vi "output.vi"(8 "error in":errorcluster, 10 "data table in":T1, 11 "OPC UA runtime in":refnum<class "OPC UA runtime.lvclass">) -> (0 "error out":errorcluster, 2 "data table out":T1, 3 "OPC UA runtime out":refnum<class "OPC UA runtime.lvclass">)   [LabVIEW 2013, in "OPC UA runtime.lvclass"]
doc: "Provides an interface for writing data to a module at runtime. While this interface performs no operations, a child should provide an override which may write to any open sessions, references, or interfaces."
uses:
  OPC UA runtime.lvclass
  <vilib>/NI/Tag Bus/table/data table.lvlib
  <vilib>/NI/Tag Bus/table/data polymorphs/read one/read Boolean.vi
  <vilib>/opcua/NI OPC UA Client.lvlib
  <vilib>/OPCUA/client/Write Bool.vi
  <vilib>/NI/Tag Bus/table/data polymorphs/read one/read I8.vi
  <vilib>/OPCUA/client/Write SByte.vi
  <vilib>/NI/Tag Bus/table/data polymorphs/read one/read U8.vi
  <vilib>/OPCUA/client/Write Byte.vi
  <vilib>/OPCUA/client/Write Int16.vi
  <vilib>/NI/Tag Bus/table/data polymorphs/read one/read I16.vi
  <vilib>/OPCUA/client/Write UInt16.vi
  <vilib>/NI/Tag Bus/table/data polymorphs/read one/read U16.vi
  <vilib>/OPCUA/client/Write Int32.vi
  <vilib>/NI/Tag Bus/table/data polymorphs/read one/read I32.vi
  <vilib>/OPCUA/client/Write UInt32.vi
  <vilib>/NI/Tag Bus/table/data polymorphs/read one/read U32.vi
  <vilib>/OPCUA/client/Write Int64.vi
  <vilib>/NI/Tag Bus/table/data polymorphs/read one/read I64.vi
  <vilib>/OPCUA/client/Write UInt64.vi
  <vilib>/NI/Tag Bus/table/data polymorphs/read one/read U64.vi
  <vilib>/OPCUA/client/Write Float.vi
  <vilib>/NI/Tag Bus/table/data polymorphs/read one/read Single.vi
  <vilib>/OPCUA/client/Write Double.vi
  <vilib>/NI/Tag Bus/table/data polymorphs/read one/read Double.vi
  <vilib>/OPCUA/client/Write String.vi
  <vilib>/NI/Tag Bus/table/data polymorphs/read one/read String.vi
  <vilib>/OPCUA/client/Write DateTime.vi
  <vilib>/OPCUA/client/Write ByteString.vi
  <vilib>/NI/Tag Bus/table/data polymorphs/read one/read Array of U8.vi
  <vilib>/OPCUA/client/Write Bool Array.vi
  <vilib>/NI/Tag Bus/table/data polymorphs/read one/read Array of Boolean.vi
  <vilib>/NI/Tag Bus/table/data polymorphs/read one/read Array of I8.vi
  <vilib>/OPCUA/client/Write SByte Array.vi
  <vilib>/OPCUA/client/Write Byte Array.vi
  <vilib>/OPCUA/client/Write Int16 Array.vi
  <vilib>/NI/Tag Bus/table/data polymorphs/read one/read Array of I16.vi
  <vilib>/OPCUA/client/Write UInt16 Array.vi
  <vilib>/NI/Tag Bus/table/data polymorphs/read one/read Array of U16.vi
  <vilib>/OPCUA/client/Write Int32 Array.vi
  <vilib>/NI/Tag Bus/table/data polymorphs/read one/read Array of I32.vi
  <vilib>/OPCUA/client/Write UInt32 Array.vi
  <vilib>/NI/Tag Bus/table/data polymorphs/read one/read Array of U32.vi
  <vilib>/OPCUA/client/Write Int64 Array.vi
  <vilib>/NI/Tag Bus/table/data polymorphs/read one/read Array of I64.vi
  <vilib>/OPCUA/client/Write UInt64 Array.vi
  <vilib>/NI/Tag Bus/table/data polymorphs/read one/read Array of U64.vi
  <vilib>/OPCUA/client/Write Float Array.vi
  <vilib>/NI/Tag Bus/table/data polymorphs/read one/read Array of Single.vi
  <vilib>/OPCUA/client/Write Double Array.vi
  <vilib>/NI/Tag Bus/table/data polymorphs/read one/read Array of Double.vi
  <vilib>/OPCUA/client/Write String Array.vi
  <vilib>/NI/Tag Bus/table/data polymorphs/read one/read Array of String.vi
  <vilib>/OPCUA/client/Write DateTime Array.vi
  <vilib>/OPCUA/client/Write ByteString Array.vi
  <vilib>/opcua/NI OPC UA Server.lvlib
  <vilib>/OPCUA/server/Write Bool.vi
  <vilib>/OPCUA/server/Write SByte.vi
  <vilib>/OPCUA/server/Write Byte.vi
  <vilib>/OPCUA/server/Write Int16.vi
  <vilib>/OPCUA/server/Write UInt16.vi
  <vilib>/OPCUA/server/Write Int32.vi
  <vilib>/OPCUA/server/Write UInt32.vi
  <vilib>/OPCUA/server/Write Int64.vi
  <vilib>/OPCUA/server/Write UInt64.vi
  <vilib>/OPCUA/server/Write Float.vi
  <vilib>/OPCUA/server/Write Double.vi
  <vilib>/OPCUA/server/Write String.vi
  <vilib>/OPCUA/server/Write Date Time.vi
  <vilib>/OPCUA/server/Write Byte String.vi
  <vilib>/OPCUA/server/Write Bool Array.vi
  <vilib>/OPCUA/server/Write SByte Array.vi
  <vilib>/OPCUA/server/Write Byte Array.vi
  <vilib>/OPCUA/server/Write Int16 Array.vi
  <vilib>/OPCUA/server/Write UInt16 Array.vi
  <vilib>/OPCUA/server/Write Int32 Array.vi
  <vilib>/OPCUA/server/Write UInt32 Array.vi
  <vilib>/OPCUA/server/Write Int64 Array.vi
  <vilib>/OPCUA/server/Write UInt64 Array.vi
  <vilib>/OPCUA/server/Write Float Array.vi
  <vilib>/OPCUA/server/Write Double Array.vi
  <vilib>/OPCUA/server/Write String Array.vi
  <vilib>/OPCUA/server/Write Date Time Array.vi
  <vilib>/OPCUA/server/Write Byte String Array.vi
  <vilib>/NI/Tag Bus/table/data table.ctl
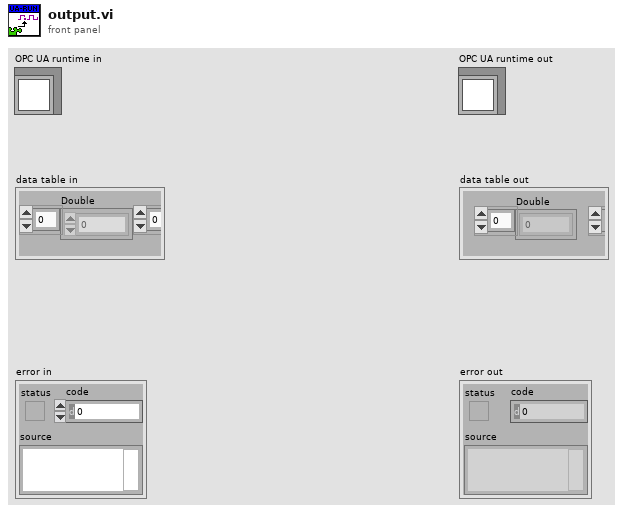
[diagram p1: front panel]
types:
  T1 = typedef "tag bus.lvlib/data table.lvlib/data table.ctl" = cluster{"Double":dbl[], "Single":sgl[], "I64":i64[], "I32":i32[], "I16":i16[], "I8":i8[], "U64":u64[], "U32":u32[], "U16":u16[], "U8":u8[], "Boolean":bool[], "String":string[], "Array of Double":cluster{"DBL Array":dbl[]}[], "Array of Single":cluster{"SGL Array":sgl[]}[], "Array of I64":cluster{"I64 Array":i64[]}[], "Array of I32":cluster{"I32 Array":i32[]}[], "Array of I16":cluster{"I16 Array":i16[]}[], "Array of I8":cluster{"I8 Array":i8[]}[], "Array of U64":cluster{"U64 Array":u64[]}[], "Array of U32":cluster{"U32 Array":u32[]}[], "Array of U16":cluster{"U16 Array":u16[]}[], "Array of U8":cluster{"U8 Array":u8[]}[], "Array of Boolean":cluster{"Boolean Array":bool[]}[], "Array of String":cluster{"String Array":string[]}[]}
  T2 = typedef "tag bus.lvlib/tag descriptor.lvclass/Data Type.ctl" = enum16{"Double", "Single", "I64", "I32", "I16", "I8", "U64", "U32", "U16", "U8", "Boolean", "String", "Array of Double", "Array of Single", "Array of I64", "Array of I32", "Array of I16", "Array of I8", "Array of U64", "Array of U32", "Array of U16", "Array of U8", "Array of Boolean", "Array of String"}
  T3 = typedef "OPC UA configuration.lvclass/OPC UA Data Type.ctl" = u16
  T4 = cluster{"DCAF Data Type":T2, "Index":i32, "Node Path":string, "OPC UA Data Type":T3}[]
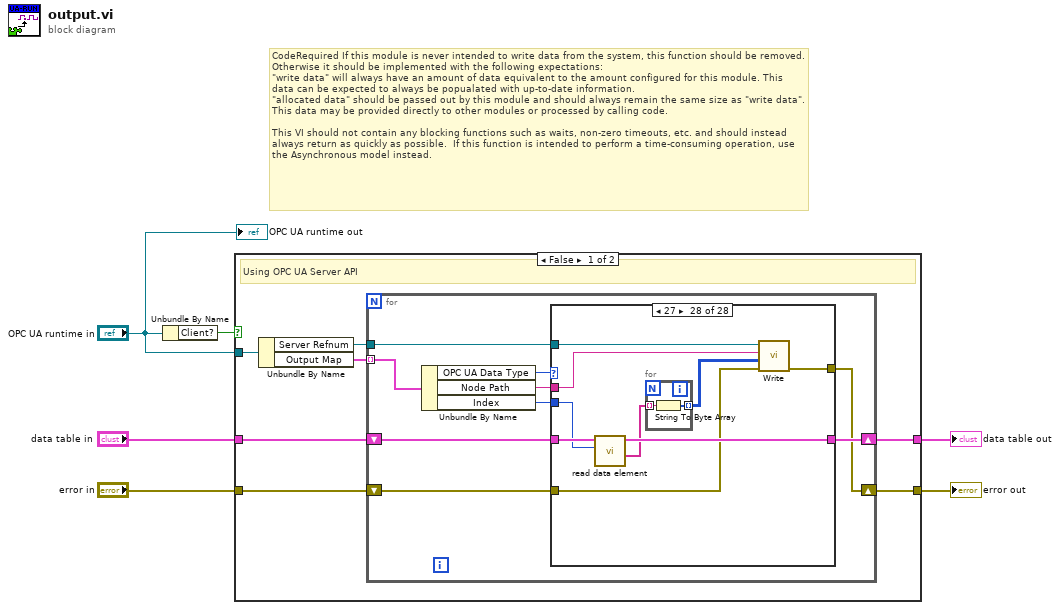
[diagram p0: block diagram]
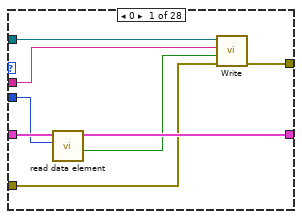
[diagram p2: hidden frame]
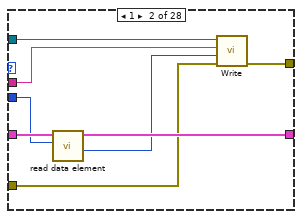
[diagram p3: hidden frame]
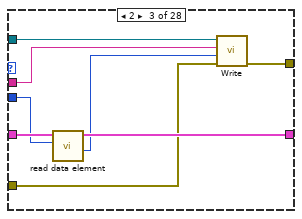
[diagram p4: hidden frame]
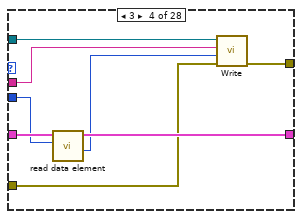
[diagram p5: hidden frame]
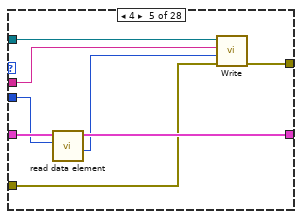
[diagram p6: hidden frame]
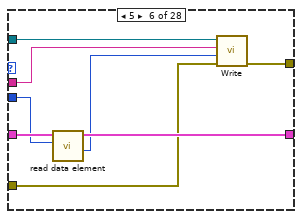
[diagram p7: hidden frame]
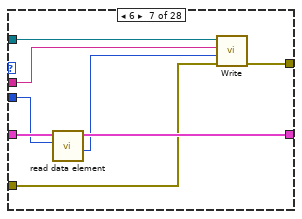
[diagram p8: hidden frame]
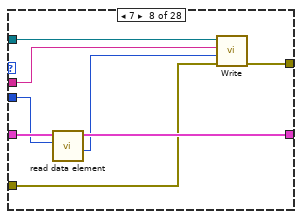
[diagram p9: hidden frame]
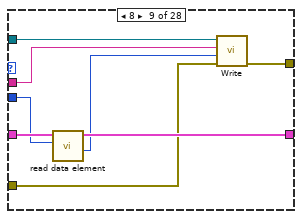
[diagram p10: hidden frame]
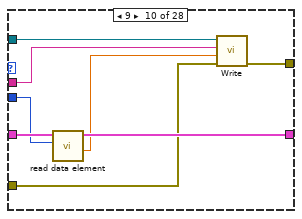
[diagram p11: hidden frame]
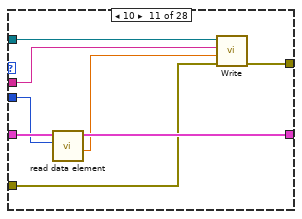
[diagram p12: hidden frame]
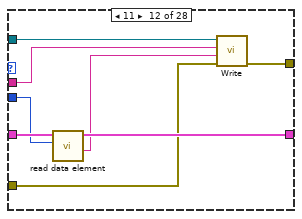
[diagram p13: hidden frame]
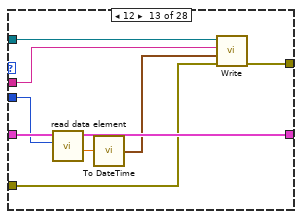
[diagram p14: hidden frame]
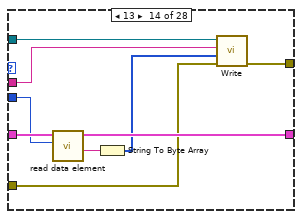
[diagram p15: hidden frame]
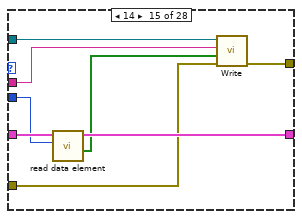
[diagram p16: hidden frame]
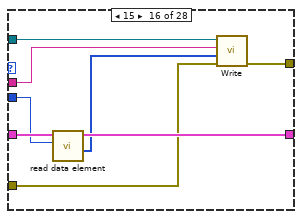
[diagram p17: hidden frame]
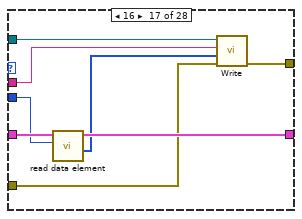
[diagram p18: hidden frame]
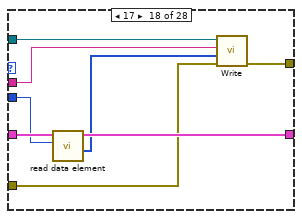
[diagram p19: hidden frame]
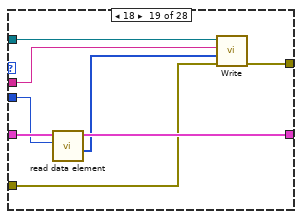
[diagram p20: hidden frame]
diagram:
  # "CodeRequired If this module is never intended to write data from the system, this function should be removed. Otherwise it should be implemented with the following expectations:\n\"write data\" will always have an amount of data equivalent to the amount configured for this module. This data can be expected to always be popualated with up-to-date information.\n\"allocated data\" should be passed out by this module and should always remain the same size as \"write data\". This data may be provided directly to other modules or processed by calling code.\n\nThis VI should not contain any blocking functions such as waits, non-zero timeouts, etc. and should instead always return as quickly as possible.  If this function is intended to perform a time-consuming operation, use the Asynchronous model instead."
  n1 = Unbundle By Name("OPC UA runtime in") -> ("Client?"=w6:bool)
  n2 = case shown="False" w6 {
    tunnel: "OPC UA runtime in" -> [w13 w259]
    tunnel: "data table in" -> [w9 w256]
    tunnel: "error in" -> [w8 w255]
    tunnel: [w10 w254] -> w2
    tunnel: [w7 w253] -> w3
    frame False {
      # "Using OPC UA Server API"
      n3 = Unbundle By Name(w13) -> ("Server Refnum"=w11:refnum<k21>, "Output Map"=w12:T4)
      n4 = for {
        tunnel: w11 -> [w16]
        tunnel: w12 -> [w22] mode=indexing
        shift-right: [w15] -> w7
        shift-left: w8 -> [w18]
        shift-right: [w19] -> w10
        shift-left: w9 -> [w20]
        n5 = Unbundle By Name(w22) -> ("OPC UA Data Type"=w21:T3, "Node Path"=w14:string, "Index"=w17:i32)
        n6 = case shown="27" w21 {
          tunnel: w20 -> [w30 w38 w46 w54 w62 w70 w78 w86 w94 w102 w110 w118 w127 w136 w144 w152 w160 w168 w176 w184 w192 w200 w208 w216 w224 w232 w241 w250]
          tunnel: [w29 w37 w45 w53 w61 w69 w77 w85 w93 w101 w109 w117 w126 w135 w143 w151 w159 w167 w175 w183 w191 w199 w207 w215 w223 w231 w240 w249] -> w19
          tunnel: w18 -> [w25 w33 w41 w49 w57 w65 w73 w81 w89 w97 w105 w113 w122 w131 w139 w147 w155 w163 w171 w179 w187 w195 w203 w211 w219 w227 w236 w245]
          tunnel: w17 -> [w28 w36 w44 w52 w60 w68 w76 w84 w92 w100 w108 w116 w125 w134 w142 w150 w158 w166 w174 w182 w190 w198 w206 w214 w222 w230 w239 w248]
          tunnel: w16 -> [w27 w35 w43 w51 w59 w67 w75 w83 w91 w99 w107 w115 w124 w133 w141 w149 w157 w165 w173 w181 w189 w197 w205 w213 w221 w229 w238 w247]
          tunnel: [w26 w34 w42 w50 w58 w66 w74 w82 w90 w98 w106 w114 w123 w132 w140 w148 w156 w164 w172 w180 w188 w196 w204 w212 w220 w228 w237 w246] -> w15
          tunnel: w14 -> [w24 w32 w40 w48 w56 w64 w72 w80 w88 w96 w104 w112 w121 w130 w138 w146 w154 w162 w170 w178 w186 w194 w202 w210 w218 w226 w235 w244]
          frame 0 {
            n7 = call-poly <vilib>:"read data element.vi"("index"=w28, "data table in"=w30) -> ("value"=w23:bool, "data table out"=w29:T1)  [unwired: 8 in]
            n8 = call-poly <vilib>:"Write.vi"("error in (no error)"=w25, "value"=w23, "node path"=w24, "OPC UA server refnum in"=w27) -> ("error out"=w26:errorcluster)  [unwired: 6 in, 1 out]
          }
          frame 1 {
            n9 = call-poly <vilib>:"read data element.vi"("index"=w36, "data table in"=w38) -> ("value"=w31:i8, "data table out"=w37:T1)  [unwired: 8 in]
            n10 = call-poly <vilib>:"Write.vi"("error in (no error)"=w33, "value"=w31, "node path"=w32, "OPC UA server refnum in"=w35) -> ("error out"=w34:errorcluster)  [unwired: 6 in, 1 out]
          }
          frame 2 {
            n11 = call-poly <vilib>:"read data element.vi"("index"=w44, "data table in"=w46) -> ("value"=w39:u8, "data table out"=w45:T1)  [unwired: 8 in]
            n12 = call-poly <vilib>:"Write.vi"("error in (no error)"=w41, "value"=w39, "node path"=w40, "OPC UA server refnum in"=w43) -> ("error out"=w42:errorcluster)  [unwired: 6 in, 1 out]
          }
          frame 3 {
            n13 = call-poly <vilib>:"read data element.vi"("index"=w52, "data table in"=w54) -> ("value"=w47:i16, "data table out"=w53:T1)  [unwired: 8 in]
            n14 = call-poly <vilib>:"Write.vi"("error in (no error)"=w49, "value"=w47, "node path"=w48, "OPC UA server refnum in"=w51) -> ("error out"=w50:errorcluster)  [unwired: 6 in, 1 out]
          }
          frame 4 {
            n15 = call-poly <vilib>:"read data element.vi"("index"=w60, "data table in"=w62) -> ("value"=w55:u16, "data table out"=w61:T1)  [unwired: 8 in]
            n16 = call-poly <vilib>:"Write.vi"("error in (no error)"=w57, "value"=w55, "node path"=w56, "OPC UA server refnum in"=w59) -> ("error out"=w58:errorcluster)  [unwired: 6 in, 1 out]
          }
          frame 5 {
            n17 = call-poly <vilib>:"read data element.vi"("index"=w68, "data table in"=w70) -> ("value"=w63:i32, "data table out"=w69:T1)  [unwired: 8 in]
            n18 = call-poly <vilib>:"Write.vi"("error in (no error)"=w65, "value"=w63, "node path"=w64, "OPC UA server refnum in"=w67) -> ("error out"=w66:errorcluster)  [unwired: 6 in, 1 out]
          }
          frame 6 {
            n19 = call-poly <vilib>:"read data element.vi"("index"=w76, "data table in"=w78) -> ("value"=w71:u32, "data table out"=w77:T1)  [unwired: 8 in]
            n20 = call-poly <vilib>:"Write.vi"("error in (no error)"=w73, "value"=w71, "node path"=w72, "OPC UA server refnum in"=w75) -> ("error out"=w74:errorcluster)  [unwired: 6 in, 1 out]
          }
          frame 7 {
            n21 = call-poly <vilib>:"read data element.vi"("index"=w84, "data table in"=w86) -> ("value"=w79:i64, "data table out"=w85:T1)  [unwired: 8 in]
            n22 = call-poly <vilib>:"Write.vi"("error in (no error)"=w81, "value"=w79, "node path"=w80, "OPC UA server refnum in"=w83) -> ("error out"=w82:errorcluster)  [unwired: 6 in, 1 out]
          }
          frame 8 {
            n23 = call-poly <vilib>:"read data element.vi"("index"=w92, "data table in"=w94) -> ("value"=w87:u64, "data table out"=w93:T1)  [unwired: 8 in]
            n24 = call-poly <vilib>:"Write.vi"("error in (no error)"=w89, "value"=w87, "node path"=w88, "OPC UA server refnum in"=w91) -> ("error out"=w90:errorcluster)  [unwired: 6 in, 1 out]
          }
          frame 9 {
            n25 = call-poly <vilib>:"read data element.vi"("index"=w100, "data table in"=w102) -> ("value"=w95:sgl, "data table out"=w101:T1)  [unwired: 8 in]
            n26 = call-poly <vilib>:"Write.vi"("error in (no error)"=w97, "value"=w95, "node path"=w96, "OPC UA server refnum in"=w99) -> ("error out"=w98:errorcluster)  [unwired: 6 in, 1 out]
          }
          frame 10 {
            n27 = call-poly <vilib>:"read data element.vi"("index"=w108, "data table in"=w110) -> ("value"=w103:dbl, "data table out"=w109:T1)  [unwired: 8 in]
            n28 = call-poly <vilib>:"Write.vi"("error in (no error)"=w105, "value"=w103, "node path"=w104, "OPC UA server refnum in"=w107) -> ("error out"=w106:errorcluster)  [unwired: 6 in, 1 out]
          }
          frame 11 {
            n29 = call-poly <vilib>:"read data element.vi"("index"=w116, "data table in"=w118) -> ("value"=w111:string, "data table out"=w117:T1)  [unwired: 8 in]
            n30 = call-poly <vilib>:"Write.vi"("error in (no error)"=w113, "value"=w111, "node path"=w112, "OPC UA server refnum in"=w115) -> ("error out"=w114:errorcluster)  [unwired: 6 in, 1 out]
          }
          frame 12 {
            n31 = call-poly <vilib>:"read data element.vi"("index"=w125, "data table in"=w127) -> ("value"=w120:dbl, "data table out"=w126:T1)  [unwired: 8 in]
            n32 = call "To DateTime.vi"("Formatted DateTime"=w120) -> ("Time Stamp"=w119:timestamp)
            n33 = call-poly <vilib>:"Write.vi"("error in (no error)"=w122, "value"=w119, "node path"=w121, "OPC UA server refnum in"=w124) -> ("error out"=w123:errorcluster)  [unwired: 6 in, 1 out]
          }
          frame 13 {
            n34 = call-poly <vilib>:"read data element.vi"("index"=w134, "data table in"=w136) -> ("value"=w129:string, "data table out"=w135:T1)  [unwired: 8 in]
            n35 = String To Byte Array(string=w129) -> (unsigned byte array=w128:u8[])
            n36 = call-poly <vilib>:"Write.vi"("error in (no error)"=w131, "value"=w128, "node path"=w130, "OPC UA server refnum in"=w133) -> ("error out"=w132:errorcluster)  [unwired: 6 in, 1 out]
          }
          frame 14 {
            n37 = call-poly <vilib>:"read data element.vi"("index"=w142, "data table in"=w144) -> ("value"=w137:bool[], "data table out"=w143:T1)  [unwired: 8 in]
            n38 = call-poly <vilib>:"Write.vi"("error in (no error)"=w139, "value"=w137, "node path"=w138, "OPC UA server refnum in"=w141) -> ("error out"=w140:errorcluster)  [unwired: 6 in, 1 out]
          }
          frame 15 {
            n39 = call-poly <vilib>:"read data element.vi"("index"=w150, "data table in"=w152) -> ("value"=w145:i8[], "data table out"=w151:T1)  [unwired: 8 in]
            n40 = call-poly <vilib>:"Write.vi"("error in (no error)"=w147, "value"=w145, "node path"=w146, "OPC UA server refnum in"=w149) -> ("error out"=w148:errorcluster)  [unwired: 6 in, 1 out]
          }
          frame 16 {
            n41 = call-poly <vilib>:"read data element.vi"("index"=w158, "data table in"=w160) -> ("value"=w153:u8[], "data table out"=w159:T1)  [unwired: 8 in]
            n42 = call-poly <vilib>:"Write.vi"("error in (no error)"=w155, "value"=w153, "node path"=w154, "OPC UA server refnum in"=w157) -> ("error out"=w156:errorcluster)  [unwired: 6 in, 1 out]
          }
          frame 17 {
            n43 = call-poly <vilib>:"read data element.vi"("index"=w166, "data table in"=w168) -> ("value"=w161:i16[], "data table out"=w167:T1)  [unwired: 8 in]
            n44 = call-poly <vilib>:"Write.vi"("error in (no error)"=w163, "value"=w161, "node path"=w162, "OPC UA server refnum in"=w165) -> ("error out"=w164:errorcluster)  [unwired: 6 in, 1 out]
          }
          frame 18 {
            n45 = call-poly <vilib>:"read data element.vi"("index"=w174, "data table in"=w176) -> ("value"=w169:u16[], "data table out"=w175:T1)  [unwired: 8 in]
            n46 = call-poly <vilib>:"Write.vi"("error in (no error)"=w171, "value"=w169, "node path"=w170, "OPC UA server refnum in"=w173) -> ("error out"=w172:errorcluster)  [unwired: 6 in, 1 out]
          }
          frame 19 {
            n47 = call-poly <vilib>:"read data element.vi"("index"=w182, "data table in"=w184) -> ("value"=w177:i32[], "data table out"=w183:T1)  [unwired: 8 in]
            n48 = call-poly <vilib>:"Write.vi"("error in (no error)"=w179, "value"=w177, "node path"=w178, "OPC UA server refnum in"=w181) -> ("error out"=w180:errorcluster)  [unwired: 6 in, 1 out]
          }
          frame 20 {
            n49 = call-poly <vilib>:"read data element.vi"("index"=w190, "data table in"=w192) -> ("value"=w185:u32[], "data table out"=w191:T1)  [unwired: 8 in]
            n50 = call-poly <vilib>:"Write.vi"("error in (no error)"=w187, "value"=w185, "node path"=w186, "OPC UA server refnum in"=w189) -> ("error out"=w188:errorcluster)  [unwired: 6 in, 1 out]
          }
          frame 21 {
            n51 = call-poly <vilib>:"read data element.vi"("index"=w198, "data table in"=w200) -> ("value"=w193:i64[], "data table out"=w199:T1)  [unwired: 8 in]
            n52 = call-poly <vilib>:"Write.vi"("error in (no error)"=w195, "value"=w193, "node path"=w194, "OPC UA server refnum in"=w197) -> ("error out"=w196:errorcluster)  [unwired: 6 in, 1 out]
          }
          frame 22 {
            n53 = call-poly <vilib>:"read data element.vi"("index"=w206, "data table in"=w208) -> ("value"=w201:u64[], "data table out"=w207:T1)  [unwired: 8 in]
            n54 = call-poly <vilib>:"Write.vi"("error in (no error)"=w203, "value"=w201, "node path"=w202, "OPC UA server refnum in"=w205) -> ("error out"=w204:errorcluster)  [unwired: 6 in, 1 out]
          }
          frame 23 {
            n55 = call-poly <vilib>:"read data element.vi"("index"=w214, "data table in"=w216) -> ("value"=w209:sgl[], "data table out"=w215:T1)  [unwired: 8 in]
            n56 = call-poly <vilib>:"Write.vi"("error in (no error)"=w211, "value"=w209, "node path"=w210, "OPC UA server refnum in"=w213) -> ("error out"=w212:errorcluster)  [unwired: 6 in, 1 out]
          }
          frame 24 {
            n57 = call-poly <vilib>:"read data element.vi"("index"=w222, "data table in"=w224) -> ("value"=w217:dbl[], "data table out"=w223:T1)  [unwired: 8 in]
            n58 = call-poly <vilib>:"Write.vi"("error in (no error)"=w219, "value"=w217, "node path"=w218, "OPC UA server refnum in"=w221) -> ("error out"=w220:errorcluster)  [unwired: 6 in, 1 out]
          }
          frame 25 {
            n59 = call-poly <vilib>:"read data element.vi"("index"=w230, "data table in"=w232) -> ("value"=w225:string[], "data table out"=w231:T1)  [unwired: 8 in]
            n60 = call-poly <vilib>:"Write.vi"("error in (no error)"=w227, "value"=w225, "node path"=w226, "OPC UA server refnum in"=w229) -> ("error out"=w228:errorcluster)  [unwired: 6 in, 1 out]
          }
          frame 26 {
            n61 = call-poly <vilib>:"read data element.vi"("index"=w239, "data table in"=w241) -> ("value"=w234:dbl[], "data table out"=w240:T1)  [unwired: 8 in]
            n62 = call "To DateTime Array.vi"("Formatted DateTime Array"=w234) -> ("DateTime Array"=w233:timestamp[])
            n63 = call-poly <vilib>:"Write.vi"("error in (no error)"=w236, "value"=w233, "node path"=w235, "OPC UA server refnum in"=w238) -> ("error out"=w237:errorcluster)  [unwired: 6 in, 1 out]
          }
          frame 27 {
            n64 = call-poly <vilib>:"read data element.vi"("index"=w248, "data table in"=w250) -> ("value"=w243:string[], "data table out"=w249:T1)  [unwired: 8 in]
            n65 = for {
              tunnel: w243 -> [w252] mode=indexing
              tunnel: [w251] -> w242 mode=indexing
              n66 = String To Byte Array(string=w252) -> (unsigned byte array=w251:u8[])
            }
            n67 = call-poly <vilib>:"Write.vi"("error in (no error)"=w245, "value"=w242, "node path"=w244, "OPC UA server refnum in"=w247) -> ("error out"=w246:errorcluster)  [unwired: 6 in, 1 out]
          }
        }
      }
    }
    frame True {
      # "Using OPC UA Client API"
      n68 = Unbundle By Name(w259) -> ("Client Refnum"=w258:refnum<k21>, "Output Map"=w257:T4)
      n69 = for {
        tunnel: w258 -> [w264]
        tunnel: w257 -> [w268] mode=indexing
        shift-right: [w261] -> w253
        shift-left: w255 -> [w263]
        shift-right: [w262] -> w254
        shift-left: w256 -> [w266]
        n70 = Unbundle By Name(w268) -> ("OPC UA Data Type"=w267:T3, "Node Path"=w260:string, "Index"=w265:i32)
        n71 = case shown="8" w267 {
          tunnel: w266 -> [w276 w284 w292 w300 w308 w316 w324 w332 w340 w348 w356 w364 w373 w382 w390 w398 w406 w414 w422 w430 w438 w446 w454 w462 w470 w478 w487 w496]
          tunnel: w265 -> [w275 w283 w291 w299 w307 w315 w323 w331 w339 w347 w355 w363 w372 w381 w389 w397 w405 w413 w421 w429 w437 w445 w453 w461 w469 w477 w486 w495]
          tunnel: w264 -> [w274 w282 w290 w298 w306 w314 w322 w330 w338 w346 w354 w362 w371 w380 w388 w396 w404 w412 w420 w428 w436 w444 w452 w460 w468 w476 w485 w494]
          tunnel: w263 -> [w273 w281 w289 w297 w305 w313 w321 w329 w337 w345 w353 w361 w370 w379 w387 w395 w403 w411 w419 w427 w435 w443 w451 w459 w467 w475 w484 w493]
          tunnel: [w272 w280 w288 w296 w304 w312 w320 w328 w336 w344 w352 w360 w369 w378 w386 w394 w402 w410 w418 w426 w434 w442 w450 w458 w466 w474 w483 w492] -> w262
          tunnel: [w271 w279 w287 w295 w303 w311 w319 w327 w335 w343 w351 w359 w368 w377 w385 w393 w401 w409 w417 w425 w433 w441 w449 w457 w465 w473 w482 w491] -> w261
          tunnel: w260 -> [w269 w277 w285 w293 w301 w309 w317 w325 w333 w341 w349 w357 w367 w376 w383 w391 w399 w407 w415 w423 w431 w439 w447 w455 w463 w471 w481 w490]
          frame 0 {
            n72 = call-poly <vilib>:"read data element.vi"("index"=w275, "data table in"=w276) -> ("value"=w270:bool, "data table out"=w272:T1)  [unwired: 8 in]
            n73 = call-poly <vilib>:"Write.vi"("error in (no error)"=w273, "value"=w270, "node path"=w269, "OPC UA client refnum in"=w274) -> ("error out"=w271:errorcluster)  [unwired: 5 in, 2 out]
          }
          frame 1 {
            n74 = call-poly <vilib>:"read data element.vi"("index"=w283, "data table in"=w284) -> ("value"=w278:i8, "data table out"=w280:T1)  [unwired: 8 in]
            n75 = call-poly <vilib>:"Write.vi"("error in (no error)"=w281, "value"=w278, "node path"=w277, "OPC UA client refnum in"=w282) -> ("error out"=w279:errorcluster)  [unwired: 5 in, 2 out]
          }
          frame 2 {
            n76 = call-poly <vilib>:"read data element.vi"("index"=w291, "data table in"=w292) -> ("value"=w286:u8, "data table out"=w288:T1)  [unwired: 8 in]
            n77 = call-poly <vilib>:"Write.vi"("error in (no error)"=w289, "value"=w286, "node path"=w285, "OPC UA client refnum in"=w290) -> ("error out"=w287:errorcluster)  [unwired: 5 in, 2 out]
          }
          frame 3 {
            n78 = call-poly <vilib>:"read data element.vi"("index"=w299, "data table in"=w300) -> ("value"=w294:i16, "data table out"=w296:T1)  [unwired: 8 in]
            n79 = call-poly <vilib>:"Write.vi"("error in (no error)"=w297, "value"=w294, "node path"=w293, "OPC UA client refnum in"=w298) -> ("error out"=w295:errorcluster)  [unwired: 5 in, 2 out]
          }
          frame 4 {
            n80 = call-poly <vilib>:"read data element.vi"("index"=w307, "data table in"=w308) -> ("value"=w302:u16, "data table out"=w304:T1)  [unwired: 8 in]
            n81 = call-poly <vilib>:"Write.vi"("error in (no error)"=w305, "value"=w302, "node path"=w301, "OPC UA client refnum in"=w306) -> ("error out"=w303:errorcluster)  [unwired: 5 in, 2 out]
          }
          frame 5 {
            n82 = call-poly <vilib>:"read data element.vi"("index"=w315, "data table in"=w316) -> ("value"=w310:i32, "data table out"=w312:T1)  [unwired: 8 in]
            n83 = call-poly <vilib>:"Write.vi"("error in (no error)"=w313, "value"=w310, "node path"=w309, "OPC UA client refnum in"=w314) -> ("error out"=w311:errorcluster)  [unwired: 5 in, 2 out]
          }
          frame 6 {
            n84 = call-poly <vilib>:"read data element.vi"("index"=w323, "data table in"=w324) -> ("value"=w318:u32, "data table out"=w320:T1)  [unwired: 8 in]
            n85 = call-poly <vilib>:"Write.vi"("error in (no error)"=w321, "value"=w318, "node path"=w317, "OPC UA client refnum in"=w322) -> ("error out"=w319:errorcluster)  [unwired: 5 in, 2 out]
          }
          frame 7 {
            n86 = call-poly <vilib>:"read data element.vi"("index"=w331, "data table in"=w332) -> ("value"=w326:i64, "data table out"=w328:T1)  [unwired: 8 in]
            n87 = call-poly <vilib>:"Write.vi"("error in (no error)"=w329, "value"=w326, "node path"=w325, "OPC UA client refnum in"=w330) -> ("error out"=w327:errorcluster)  [unwired: 5 in, 2 out]
          }
          frame 8 {
            n88 = call-poly <vilib>:"read data element.vi"("index"=w339, "data table in"=w340) -> ("value"=w334:u64, "data table out"=w336:T1)  [unwired: 8 in]
            n89 = call-poly <vilib>:"Write.vi"("error in (no error)"=w337, "value"=w334, "node path"=w333, "OPC UA client refnum in"=w338) -> ("error out"=w335:errorcluster)  [unwired: 5 in, 2 out]
          }
          frame 9 {
            n90 = call-poly <vilib>:"read data element.vi"("index"=w347, "data table in"=w348) -> ("value"=w342:sgl, "data table out"=w344:T1)  [unwired: 8 in]
            n91 = call-poly <vilib>:"Write.vi"("error in (no error)"=w345, "value"=w342, "node path"=w341, "OPC UA client refnum in"=w346) -> ("error out"=w343:errorcluster)  [unwired: 5 in, 2 out]
          }
          frame 10 {
            n92 = call-poly <vilib>:"read data element.vi"("index"=w355, "data table in"=w356) -> ("value"=w350:dbl, "data table out"=w352:T1)  [unwired: 8 in]
            n93 = call-poly <vilib>:"Write.vi"("error in (no error)"=w353, "value"=w350, "node path"=w349, "OPC UA client refnum in"=w354) -> ("error out"=w351:errorcluster)  [unwired: 5 in, 2 out]
          }
          frame 11 {
            n94 = call-poly <vilib>:"read data element.vi"("index"=w363, "data table in"=w364) -> ("value"=w358:string, "data table out"=w360:T1)  [unwired: 8 in]
            n95 = call-poly <vilib>:"Write.vi"("error in (no error)"=w361, "value"=w358, "node path"=w357, "OPC UA client refnum in"=w362) -> ("error out"=w359:errorcluster)  [unwired: 5 in, 2 out]
          }
          frame 12 {
            n96 = call-poly <vilib>:"read data element.vi"("index"=w372, "data table in"=w373) -> ("value"=w366:dbl, "data table out"=w369:T1)  [unwired: 8 in]
            n97 = call "To DateTime.vi"("Formatted DateTime"=w366) -> ("Time Stamp"=w365:timestamp)
            n98 = call-poly <vilib>:"Write.vi"("error in (no error)"=w370, "value"=w365, "node path"=w367, "OPC UA client refnum in"=w371) -> ("error out"=w368:errorcluster)  [unwired: 5 in, 2 out]
          }
          frame 13 {
            n99 = call-poly <vilib>:"read data element.vi"("index"=w381, "data table in"=w382) -> ("value"=w375:string, "data table out"=w378:T1)  [unwired: 8 in]
            n100 = String To Byte Array(string=w375) -> (unsigned byte array=w374:u8[])
            n101 = call-poly <vilib>:"Write.vi"("error in (no error)"=w379, "value"=w374, "node path"=w376, "OPC UA client refnum in"=w380) -> ("error out"=w377:errorcluster)  [unwired: 5 in, 2 out]
          }
          frame 14 {
            n102 = call-poly <vilib>:"read data element.vi"("index"=w389, "data table in"=w390) -> ("value"=w384:bool[], "data table out"=w386:T1)  [unwired: 8 in]
            n103 = call-poly <vilib>:"Write.vi"("error in (no error)"=w387, "value"=w384, "node path"=w383, "OPC UA client refnum in"=w388) -> ("error out"=w385:errorcluster)  [unwired: 5 in, 2 out]
          }
          frame 15 {
            n104 = call-poly <vilib>:"read data element.vi"("index"=w397, "data table in"=w398) -> ("value"=w392:i8[], "data table out"=w394:T1)  [unwired: 8 in]
            n105 = call-poly <vilib>:"Write.vi"("error in (no error)"=w395, "value"=w392, "node path"=w391, "OPC UA client refnum in"=w396) -> ("error out"=w393:errorcluster)  [unwired: 5 in, 2 out]
          }
          frame 16 {
            n106 = call-poly <vilib>:"read data element.vi"("index"=w405, "data table in"=w406) -> ("value"=w400:u8[], "data table out"=w402:T1)  [unwired: 8 in]
            n107 = call-poly <vilib>:"Write.vi"("error in (no error)"=w403, "value"=w400, "node path"=w399, "OPC UA client refnum in"=w404) -> ("error out"=w401:errorcluster)  [unwired: 5 in, 2 out]
          }
          frame 17 {
            n108 = call-poly <vilib>:"read data element.vi"("index"=w413, "data table in"=w414) -> ("value"=w408:i16[], "data table out"=w410:T1)  [unwired: 8 in]
            n109 = call-poly <vilib>:"Write.vi"("error in (no error)"=w411, "value"=w408, "node path"=w407, "OPC UA client refnum in"=w412) -> ("error out"=w409:errorcluster)  [unwired: 5 in, 2 out]
          }
          frame 18 {
            n110 = call-poly <vilib>:"read data element.vi"("index"=w421, "data table in"=w422) -> ("value"=w416:u16[], "data table out"=w418:T1)  [unwired: 8 in]
            n111 = call-poly <vilib>:"Write.vi"("error in (no error)"=w419, "value"=w416, "node path"=w415, "OPC UA client refnum in"=w420) -> ("error out"=w417:errorcluster)  [unwired: 5 in, 2 out]
          }
          frame 19 {
            n112 = call-poly <vilib>:"read data element.vi"("index"=w429, "data table in"=w430) -> ("value"=w424:i32[], "data table out"=w426:T1)  [unwired: 8 in]
            n113 = call-poly <vilib>:"Write.vi"("error in (no error)"=w427, "value"=w424, "node path"=w423, "OPC UA client refnum in"=w428) -> ("error out"=w425:errorcluster)  [unwired: 5 in, 2 out]
          }
          frame 20 {
            n114 = call-poly <vilib>:"read data element.vi"("index"=w437, "data table in"=w438) -> ("value"=w432:u32[], "data table out"=w434:T1)  [unwired: 8 in]
            n115 = call-poly <vilib>:"Write.vi"("error in (no error)"=w435, "value"=w432, "node path"=w431, "OPC UA client refnum in"=w436) -> ("error out"=w433:errorcluster)  [unwired: 5 in, 2 out]
          }
          frame 21 {
            n116 = call-poly <vilib>:"read data element.vi"("index"=w445, "data table in"=w446) -> ("value"=w440:i64[], "data table out"=w442:T1)  [unwired: 8 in]
            n117 = call-poly <vilib>:"Write.vi"("error in (no error)"=w443, "value"=w440, "node path"=w439, "OPC UA client refnum in"=w444) -> ("error out"=w441:errorcluster)  [unwired: 5 in, 2 out]
          }
          frame 22 {
            n118 = call-poly <vilib>:"read data element.vi"("index"=w453, "data table in"=w454) -> ("value"=w448:u64[], "data table out"=w450:T1)  [unwired: 8 in]
            n119 = call-poly <vilib>:"Write.vi"("error in (no error)"=w451, "value"=w448, "node path"=w447, "OPC UA client refnum in"=w452) -> ("error out"=w449:errorcluster)  [unwired: 5 in, 2 out]
          }
          frame 23 {
            n120 = call-poly <vilib>:"read data element.vi"("index"=w461, "data table in"=w462) -> ("value"=w456:sgl[], "data table out"=w458:T1)  [unwired: 8 in]
            n121 = call-poly <vilib>:"Write.vi"("error in (no error)"=w459, "value"=w456, "node path"=w455, "OPC UA client refnum in"=w460) -> ("error out"=w457:errorcluster)  [unwired: 5 in, 2 out]
          }
          frame 24 {
            n122 = call-poly <vilib>:"read data element.vi"("index"=w469, "data table in"=w470) -> ("value"=w464:dbl[], "data table out"=w466:T1)  [unwired: 8 in]
            n123 = call-poly <vilib>:"Write.vi"("error in (no error)"=w467, "value"=w464, "node path"=w463, "OPC UA client refnum in"=w468) -> ("error out"=w465:errorcluster)  [unwired: 5 in, 2 out]
          }
          frame 25 {
            n124 = call-poly <vilib>:"read data element.vi"("index"=w477, "data table in"=w478) -> ("value"=w472:string[], "data table out"=w474:T1)  [unwired: 8 in]
            n125 = call-poly <vilib>:"Write.vi"("error in (no error)"=w475, "value"=w472, "node path"=w471, "OPC UA client refnum in"=w476) -> ("error out"=w473:errorcluster)  [unwired: 5 in, 2 out]
          }
          frame 26 {
            n126 = call-poly <vilib>:"read data element.vi"("index"=w486, "data table in"=w487) -> ("value"=w480:dbl[], "data table out"=w483:T1)  [unwired: 8 in]
            n127 = call "To DateTime Array.vi"("Formatted DateTime Array"=w480) -> ("DateTime Array"=w479:timestamp[])
            n128 = call-poly <vilib>:"Write.vi"("error in (no error)"=w484, "value"=w479, "node path"=w481, "OPC UA client refnum in"=w485) -> ("error out"=w482:errorcluster)  [unwired: 5 in, 2 out]
          }
          frame 27 {
            n129 = call-poly <vilib>:"read data element.vi"("index"=w495, "data table in"=w496) -> ("value"=w489:string[], "data table out"=w492:T1)  [unwired: 8 in]
            n130 = for {
              tunnel: w489 -> [w498] mode=indexing
              tunnel: [w497] -> w488 mode=indexing
              n131 = String To Byte Array(string=w498) -> (unsigned byte array=w497:u8[])
            }
            n132 = call-poly <vilib>:"Write.vi"("error in (no error)"=w493, "value"=w488, "node path"=w490, "OPC UA client refnum in"=w494) -> ("error out"=w491:errorcluster)  [unwired: 5 in, 2 out]
          }
        }
      }
    }
  }
  "error out" <- w3
  "data table out" <- w2
  "OPC UA runtime out" <- "OPC UA runtime in"
